vi "UI Switch.vi"(8 "error in (no error)":errorcluster, 11 "UI_Top_Customer in":refnum<class "UI_Top_Customer.lvclass">) -> (0 "error out":errorcluster, 3 "UI_Top_Customer out":refnum<class "UI_Top_Customer.lvclass">)   [LabVIEW 2021, in "UI_Top_Customer.lvclass"]
uses:
  UI_Top_Customer.lvclass
  C:/Program Files (x86)/National Instruments/LabVIEW 2021/user.lib/John_Lib/AbstractActorTemplate/AbstractActorTemplate/UIActorTop.lvclass
  UI_Top_Customer.lvclass/UI_Top_Customer.ctl
  <userlib>/John_Lib/Control/Panel State.ctl
  <vilib>/Utility/miscctls.llb/LVRectTypeDef.ctl
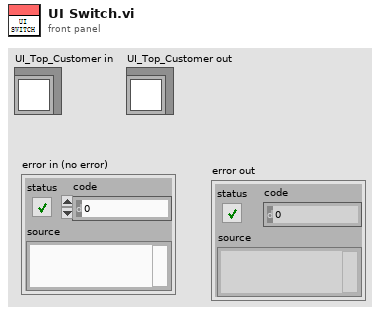
[diagram p1: front panel]
types:
  T1 = typedef "LVRectTypeDef.ctl" = cluster{"Left":i16, "Top":i16, "Right":i16, "Bottom":i16}
  T2 = enum32{"Invalid", "Standard", "Closed", "Hidden", "Minimized", "Maximized"}
  T3 = typedef "Panel State.ctl" = string
  T4 = typedef "LVAllMonitorsDisplayTypeDef.ctl" = cluster{"Bounds":cluster{"Left":i16, "Top":i16, "Right":i16, "Bottom":i16}, "Depth":i16}[]
  T5 = cluster{"Bounds":cluster{"Left":i16, "Top":i16, "Right":i16, "Bottom":i16}, "Depth":i16}
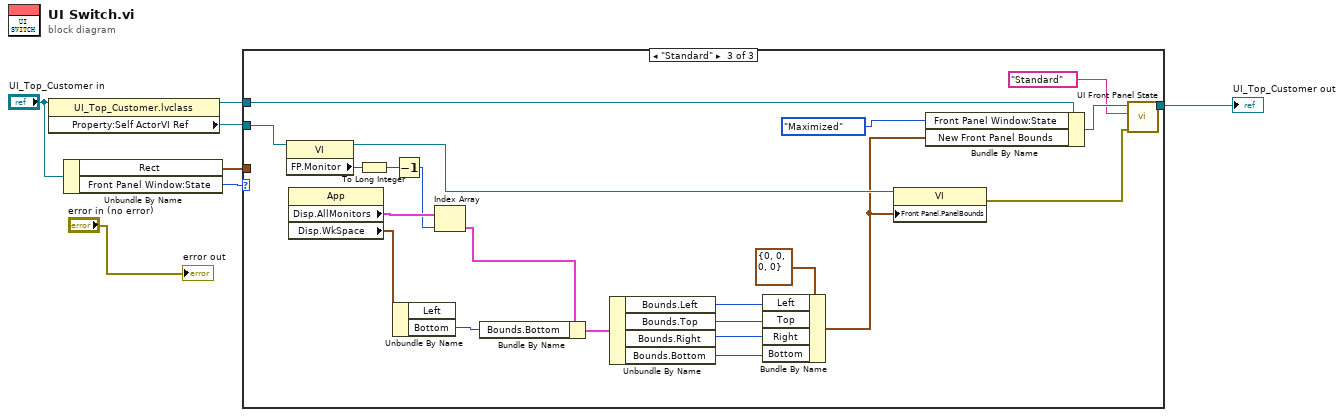
[diagram p0: block diagram]
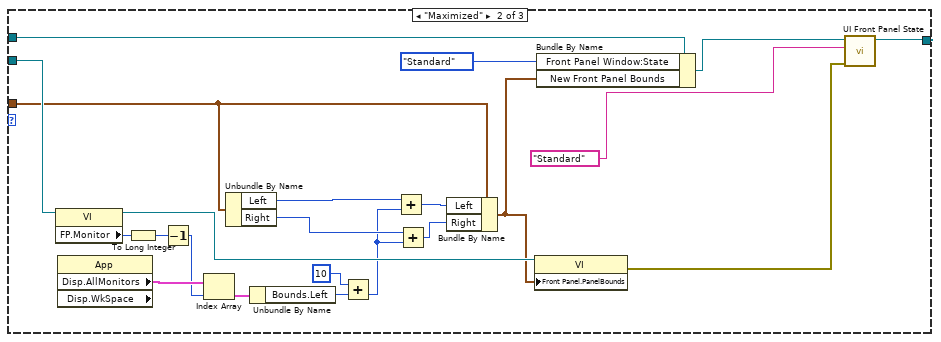
[diagram p3: hidden frame]
diagram:
  n1 = property class="UI_Top_Customer.lvclass"(reference="UI_Top_Customer in") -> (reference out=w3:refnum<class "UI_Top_Customer.lvclass">, "Property:Self ActorVI Ref"=w4:refnum<vi>)  [unwired: 1 in, 1 out]
  n2 = Unbundle By Name("UI_Top_Customer in") -> ("Rect"=w5:T1, "Front Panel Window:State"=w6:T2)
  n3 = case shown="\"Standard\"" w6 {
    tunnel: w3 -> [w8 w29 w51]
    tunnel: [w8 w9 w31] -> w2
    tunnel: w4 -> [_ w24 w46]
    tunnel: w5 -> [_ w23 _]
    frame "Invalid", Default {
    }
    frame "Maximized" {
      n4 = property class="VI"(reference=w24) -> (reference out=w18:refnum<vi>, "FP.Monitor"=w27:u16)  [unwired: 1 in, 1 out]
      n5 = property class="App" props=["Disp.AllMonitors", "Disp.WkSpace"]() -> ("Disp.AllMonitors"=w28:T4)  [unwired: 2 in, 3 out]
      n6 = To Long Integer(number=w27) -> (32bit integer=w25:i32)
      n7 = Decrement(x=w25) -> (x-1=w26:i32)
      n8 = Index Array(array=w28, index=w26) -> (element=w22:T5)
      n9 = Unbundle By Name(w23) -> ("Left"=w21:i16, "Right"=w20:i16)
      n10 = Unbundle By Name(w22) -> ("Bounds.Left"=w19:i16)
      n11 = Add(x=i16 10, y=w19) -> (x+y=w15:i16)
      n12 = Add(x=w21, y=w15) -> (x+y=w17:i16)
      n13 = Add(x=w20, y=w15) -> (x+y=w16:i16)
      n14 = Bundle By Name(cluster=w23, "Left"=w17, "Right"=w16) -> (w13:T1)
      n15 = property class="VI"(reference=w18, "Front Panel.PanelBounds"=w13) -> (error out=w12:errorcluster)  [unwired: 1 in, 1 out]
      n16 = Bundle By Name(cluster=w29, "Front Panel Window:State"=T2."Standard", "New Front Panel Bounds"=w13) -> (w10:refnum<class "UI_Top_Customer.lvclass">)
      n17 = call-dynamic "UI Front Panel State.vi"("error in (no error)"=w12, "Argument"=T3 "Standard", "UI ActorTop in"=w10) -> ("UI ActorTop out"=w9:refnum<class "UI_Top_Customer.lvclass">)  [unwired: 7 in, 1 out]
    }
    frame "Standard" {
      n18 = property class="VI"(reference=w46) -> (reference out=w45:refnum<vi>, "FP.Monitor"=w49:u16)  [unwired: 1 in, 1 out]
      n19 = property class="App"() -> ("Disp.AllMonitors"=w50:T4, "Disp.WkSpace"=w43:T1)  [unwired: 2 in, 2 out]
      n20 = To Long Integer(number=w49) -> (32bit integer=w47:i32)
      n21 = Unbundle By Name(w43) -> ("Bottom"=w42:i16)  [unwired: 1 out]
      n22 = Decrement(x=w47) -> (x-1=w48:i32)
      n23 = Index Array(array=w50, index=w48) -> (element=w44:T5)
      n24 = Bundle By Name(cluster=w44, "Bounds.Bottom"=w42) -> (w40:T5)
      n25 = Unbundle By Name(w40) -> ("Bounds.Left"=w39:i16, "Bounds.Top"=w38:i16, "Bounds.Right"=w37:i16, "Bounds.Bottom"=w36:i16)
      n26 = Bundle By Name(cluster=T1 {"Left"=0, "Top"=0, "Right"=0, "Bottom"=0} ("Front Panel Window:Panel Bounds"), "Left"=w39, "Top"=w38, "Right"=w37, "Bottom"=w36) -> (w35:T1)
      n27 = property class="VI"(reference=w45, "Front Panel.PanelBounds"=w35) -> (error out=w32:errorcluster)  [unwired: 1 in, 1 out]
      n28 = Bundle By Name(cluster=w51, "Front Panel Window:State"=T2."Maximized", "New Front Panel Bounds"=w35) -> (w34:refnum<class "UI_Top_Customer.lvclass">)
      n29 = call-dynamic "UI Front Panel State.vi"("error in (no error)"=w32, "Argument"=T3 "Standard", "UI ActorTop in"=w34) -> ("UI ActorTop out"=w31:refnum<class "UI_Top_Customer.lvclass">)  [unwired: 7 in, 1 out]
    }
  }
  "UI_Top_Customer out" <- w2
  "error out" <- "error in (no error)"
